vi "edit_entry.vi"(4 "Converted":dbl[](array[numeric]), 5 "Average":dbl, 6 "Raw":dbl[](array[numeric]), 7 "Offset":dbl, 8 "error in":errorcluster, 9 "size(s)":i32, 10 "Label":string, 11 "Active Analog Data In":T1[](array[typedef])) -> (0 "error out":errorcluster, 1 "Found?":bool, 3 "Active Analog Data Out":T1[](array[typedef]))   [LabVIEW 2017]
uses:
  analog_data.ctl
panel:
  in  "Analog Data":T1
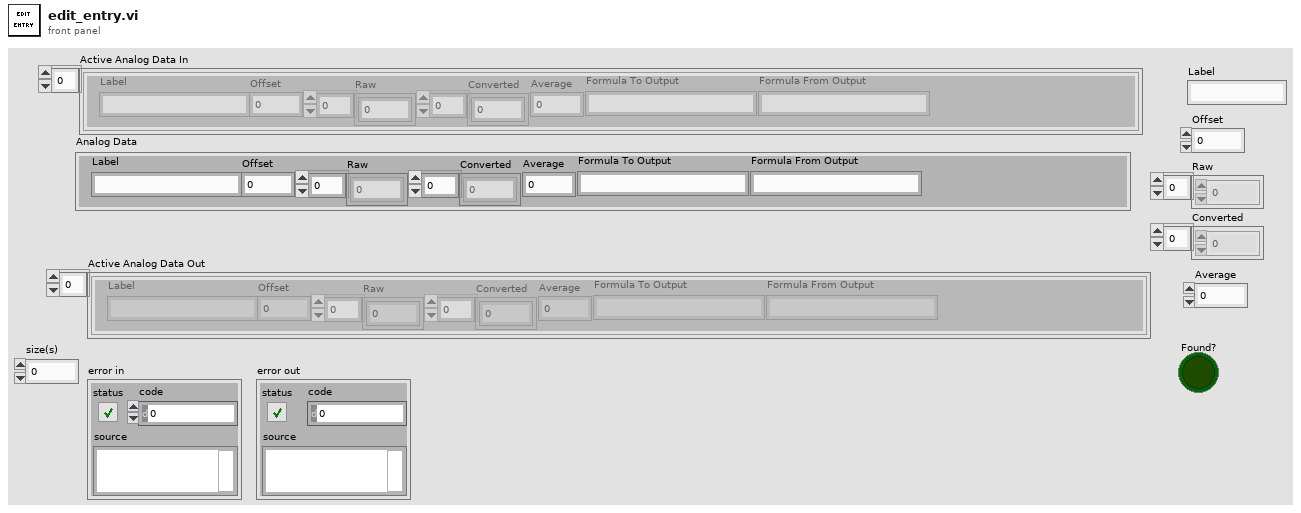
[diagram p1: front panel]
types:
  T1 = typedef "analog_data.ctl" = cluster{"Label":string, "Offset":dbl, "Raw":dbl[], "Converted":dbl[], "Average":dbl, "Formula To Output":string, "Formula From Output":string}
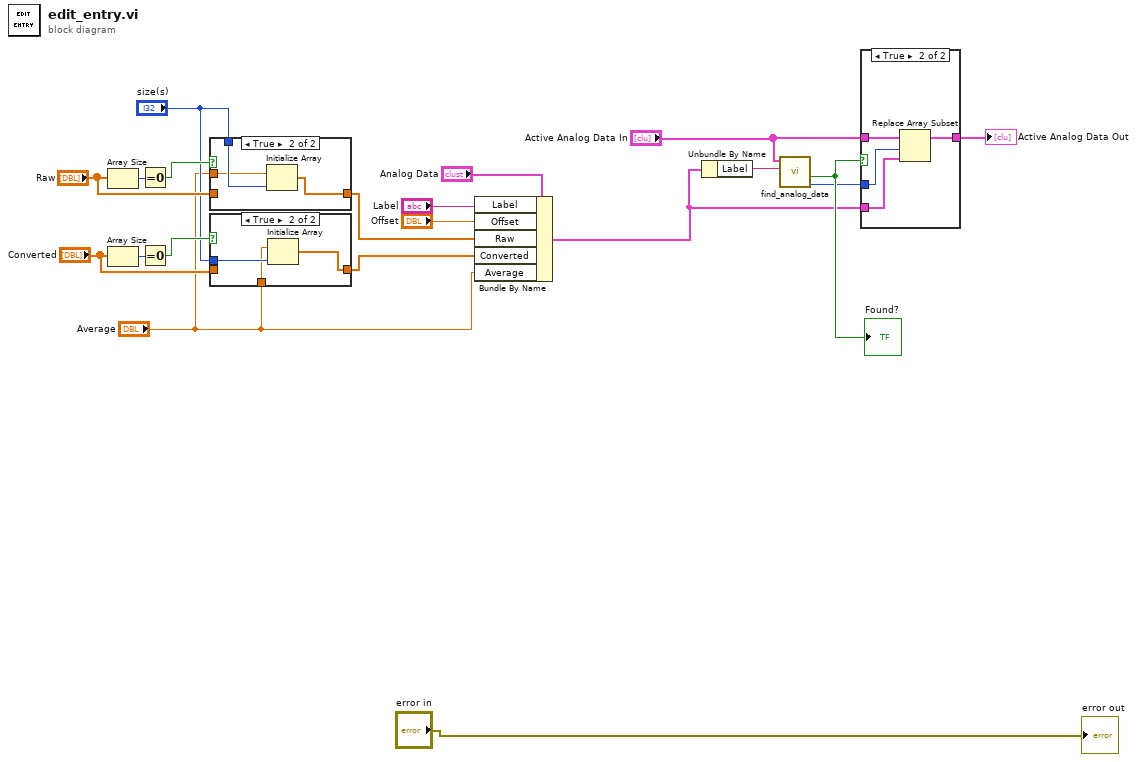
[diagram p0: block diagram]
diagram:
  n1 = Array Size(array="Raw") -> (size(s)=w10:i32)
  n2 = Array Size(array="Converted") -> (size(s)=w6:i32)
  n3 = Equal To 0?(x=w10) -> (x = 0?=w9:bool)
  n4 = Equal To 0?(x=w6) -> (x = 0?=w5:bool)
  n5 = case shown="True" w9 {
    tunnel: "Raw" -> [w21 _]
    tunnel: [w21 w22] -> w7
    tunnel: "size(s)" -> [_ w24]
    tunnel: "Average" -> [_ w23]
    frame False {
    }
    frame True {
      n6 = Initialize Array(w23, w24) -> (w22:dbl[])
    }
  }
  n7 = case shown="True" w5 {
    tunnel: "Converted" -> [w25 _]
    tunnel: [w25 w26] -> w3
    tunnel: "size(s)" -> [_ w28]
    tunnel: "Average" -> [_ w27]
    frame False {
    }
    frame True {
      n8 = Initialize Array(w27, w28) -> (w26:dbl[])
    }
  }
  n9 = Bundle By Name(cluster="Analog Data", "Label"="Label", "Offset"="Offset", "Raw"=w7, "Converted"=w3, "Average"="Average") -> (w13:T1)
  n10 = Unbundle By Name(w13) -> ("Label"=w17:string)
  n11 = call "find_analog_data.vi"("Needle"=w17, "Haystack"="Active Analog Data In") -> ("Index"=w15:i32, "Found?"=w16:bool)  [unwired: 7 in, 1 out]
  "Found?" <- w16
  n12 = case shown="True" w16 {
    tunnel: [w29 w33] -> w20
    tunnel: "Active Analog Data In" -> [w29 w32]
    tunnel: w13 -> [_ w31]
    tunnel: w15 -> [_ w30]
    frame False {
    }
    frame True {
      n13 = Replace Array Subset(array=w32, new element=w31, index=w30) -> (w33:T1[])
    }
  }
  "Active Analog Data Out" <- w20
  "error out" <- "error in"
